vi "Write Parameters.vi"(8 "error in (no error)":errorcluster, 10 "Parameters":variant, 11 "Mag Lab Parameters in":refnum<class "Mag Lab Parameters.lvclass">) -> (0 "error out":errorcluster, 3 "Mag Lab Parameters out":refnum<class "Mag Lab Parameters.lvclass">)   [LabVIEW 2015, in "Mag Lab Parameters.lvclass"]
uses:
  Mag Lab Parameters.lvclass
  Mag Lab Parameters.lvclass/Mag Lab Parameters.ctl
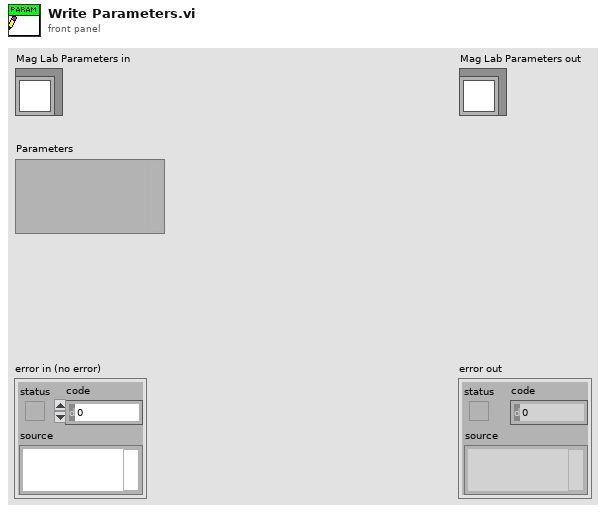
[diagram p1: front panel]
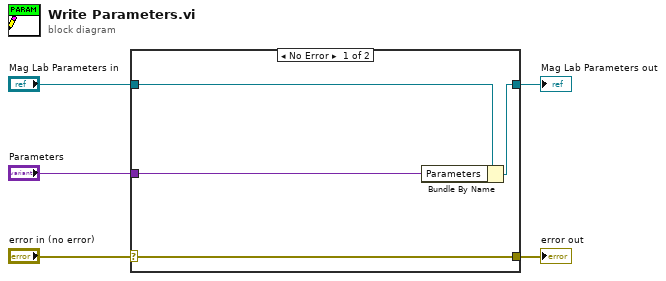
[diagram p0: block diagram]
diagram:
  n1 = case shown="No Error" "error in (no error)" {
    selector: "error in (no error)" -> [w9 w10]
    tunnel: [w9 w10] -> w4
    tunnel: [w7 w11] -> w2
    tunnel: "Mag Lab Parameters in" -> [w8 w11]
    tunnel: "Parameters" -> [w6 _]
    frame No Error {
      n2 = Bundle By Name(cluster=w8, "Parameters"=w6) -> (w7:refnum<class "Mag Lab Parameters.lvclass">)
    }
    frame Error {
    }
  }
  "error out" <- w4
  "Mag Lab Parameters out" <- w2
